vi "Execute.vi"(8 "error in (no error)":errorcluster, 10 "Cmd Data":variant, 11 "YActor in":refnum<class>) -> (0 "error out":errorcluster, 2 "Reply Data":variant, 3 "YActor out":refnum<class>, 4 "Exit":bool)   [LabVIEW 2021, in "YActor.lvclass"]
uses:
  YActor.lvclass
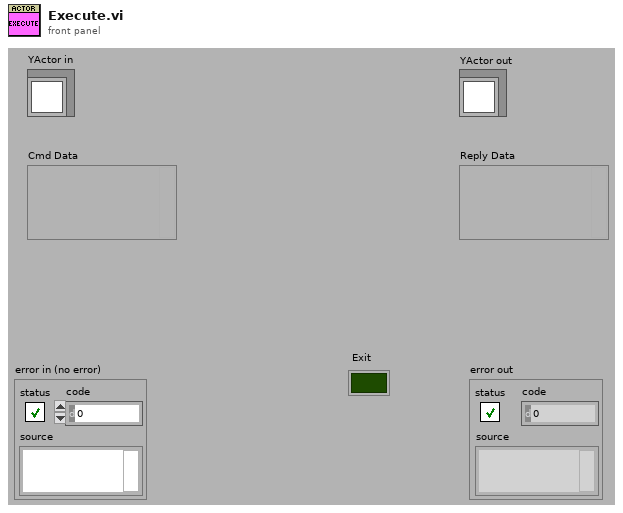
[diagram p1: front panel]
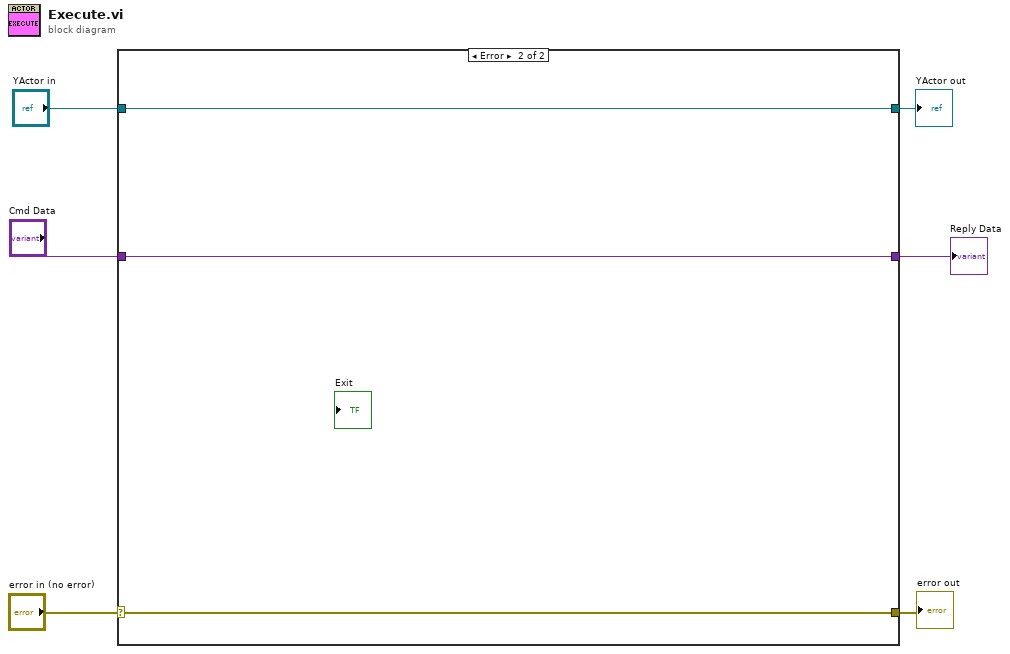
[diagram p0: block diagram]
diagram:
  n1 = case shown="Error" "error in (no error)" {
    selector: "error in (no error)" -> [w8 w12]
    tunnel: [w8 w12] -> w5
    tunnel: [w9 w11] -> w3
    tunnel: "YActor in" -> [w9 w11]
    tunnel: "Cmd Data" -> [w7 w10]
    tunnel: [w7 w10] -> w2
    frame No Error {
    }
    frame Error {
    }
  }
  "error out" <- w5
  "YActor out" <- w3
  "Reply Data" <- w2
